vi "normalize128_motor.vi"(4 "D":dbl, 5 "C":dbl, 6 "B":dbl, 7 "A":dbl) -> (0 "mD":dbl, 1 "mC":dbl, 2 "mB":dbl, 3 "mA":dbl)   [LabVIEW 2010, in "LASA Beta.lvrbt"]
doc: "Converts the FTC Controller (values from -127 to 127) to a LEGO/TETRIX readable motor value from -100 to 100."
uses:
  LASA Beta.lvrbt
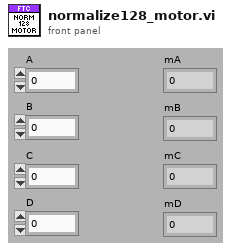
[diagram p1: front panel]
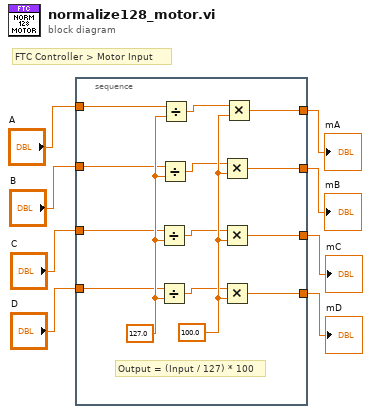
[diagram p0: block diagram]
diagram:
  # "FTC Controller > Motor Input"
  n1 = stacked-sequence {
    tunnel: "A" -> [w16]
    tunnel: [w15] -> w7
    tunnel: "B" -> [w14]
    tunnel: [w13] -> w5
    tunnel: "C" -> [w12]
    tunnel: [w11] -> w3
    tunnel: "D" -> [w10]
    tunnel: [w9] -> w1
    frame #0 {
      w21 = 100.0 ("y")
      w22 = 127.0 ("y")
      # "Output = (Input / 127) * 100"
      n2 = Divide(x=w12, y=w22) -> (x/y=w18:dbl)
      n3 = Divide(x=w10, y=w22) -> (x/y=w17:dbl)
      n4 = Divide(x=w14, y=w22) -> (x/y=w19:dbl)
      n5 = Divide(x=w16, y=w22) -> (x/y=w20:dbl)
      n6 = Multiply(x=w19, y=w21) -> (x*y=w13:dbl)
      n7 = Multiply(x=w18, y=w21) -> (x*y=w11:dbl)
      n8 = Multiply(x=w17, y=w21) -> (x*y=w9:dbl)
      n9 = Multiply(x=w20, y=w21) -> (x*y=w15:dbl)
    }
  }
  "mA" <- w7
  "mB" <- w5
  "mC" <- w3
  "mD" <- w1
